vi "2 MissionSetpoints.vi"() -> (3 "Setpoints Out":T1)   [LabVIEW 2011]
doc: "The MissionSetpoints VI determines the best sail and rudder setpoints to get to the current goal. Currently it implements a simple system based off of a series of waypoints that points the bow of the ship in the direction of the next waypoint."
uses:
  2 Typedefs/setpoints to arbiter.ctl
  2 Classes/MissionQueue/MissionQueue.lvclass
panel:
  out "Optimal Heading":dbl
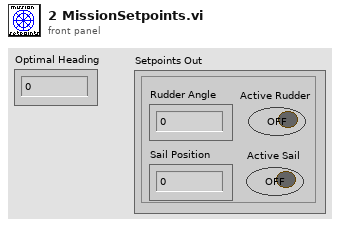
[diagram p1: front panel]
types:
  T1 = typedef "setpoints to arbiter.ctl" = cluster{"Rudder Angle":dbl, "Sail Position":dbl, "Active Rudder":bool, "Active Sail":bool}
  T2 = typedef "sail setpt.ctl" = dbl
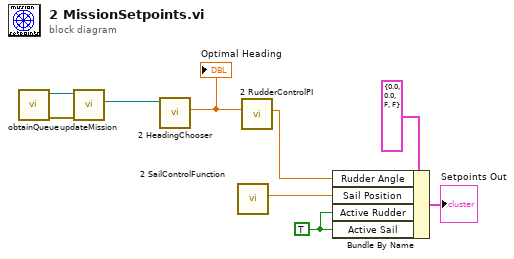
[diagram p0: block diagram]
diagram:
  w4 = TRUE
  n1 = call "obtainQueue.vi"() -> ("Error Out"=w8:errorcluster, "MissionQueue.lvclass"=w9:refnum<class "MissionQueue.lvclass">)  [unwired: 10 in]
  n2 = call "updateMission.vi"("error in (no error)"=w8, "MissionQueue in"=w9) -> ("CurrentMission"=w1:refnum<class "GenericMission.lvclass">)  [unwired: 7 in, 2 out]
  n3 = call "2 HeadingChooser.vi"("CurrentMission"=w1) -> ("Optimal Heading Out"=w2:dbl)  [unwired: 9 in, 1 out]
  "Optimal Heading" <- w2
  n4 = call "2 SailControlFunction.vi"() -> ("Sail Position"=w5:T2)  [unwired: 11 in]
  n5 = call "2 RudderControlPI.vi"("Desired Heading"=w2) -> ("Rudder Output"=w3:dbl)  [unwired: 10 in]
  n6 = Bundle By Name(cluster=T1 {"Rudder Angle"=0.0, "Sail Position"=0.0, "Active Rudder"=FALSE, "Active Sail"=FALSE} ("Setpoints Out"), "Rudder Angle"=w3, "Sail Position"=w5, "Active Rudder"=w4, "Active Sail"=w4) -> (→"Setpoints Out":T1)
